vi "WSVCAP SHL Host LL SPI Write Read.vi"(0 "SPI Data [DUT Ordered]":u8[][](array[numeric]) format="%.0x", 1 "Wait Ticks":u32, 5 "Socket Mask":u16=1 format="%02x", 7 "Cycle CMD Lengths Out (bits)":u8[](array[numeric]), 9 "Cycle CMD Delay Out (ticks)":u32[](array[numeric]), 11 "error in":errorcluster) -> (4 "SPI Read Data [DUT Ordered]":u8[][](array[numeric]), 8 "Status":u8[](array[numeric]), 15 "error out":errorcluster)   [LabVIEW 2012]
uses:
  Type Defs/WSVCAP SHL Top Level Write Read State Enum.ctl
  Type Defs/WSVCAP SHL State.ctl
  Type Defs/WSVCAP SHL Top Level Control Enum.ctl
panel:
  out "Bit Array":u32[](array[numeric]) format="%.0x"
  out "Write Data":u64[](array[numeric]) format="%032b"
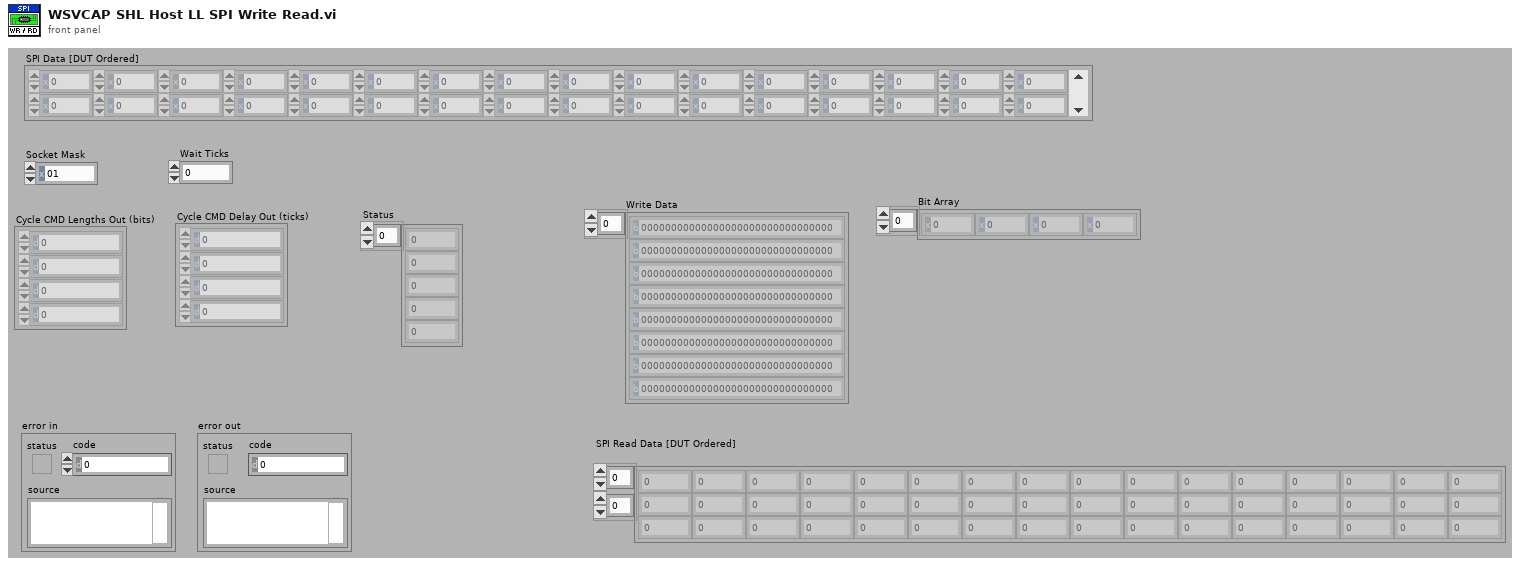
[diagram p1: front panel]
types:
  T1 = typedef "WSVCAP SHL Top Level Write Read State Enum.ctl" = enum16{"Start", "Write", "Read", "Get Status", "Wait Until Done"}
  T2 = typedef "WSVCAP SHL State.ctl" = enum8{"Idle", "Transfer Data"}
  T3 = typedef "WSVCAP SHL Top Level Control Enum.ctl" = enum16{"Start", "Cmd", "Transaction", "Wait Ticks", "Socket Mask", "Slave Address", "Sub Address", "Bytes to Write", "Bytes to Read", "Write Data", "Write Flag", "Read Data", "Read Flag", "Ack Read", "Read Status Flag", "Ack Read Status", "Status", "Cycle Count", "Stop Cycle", "Exit"}
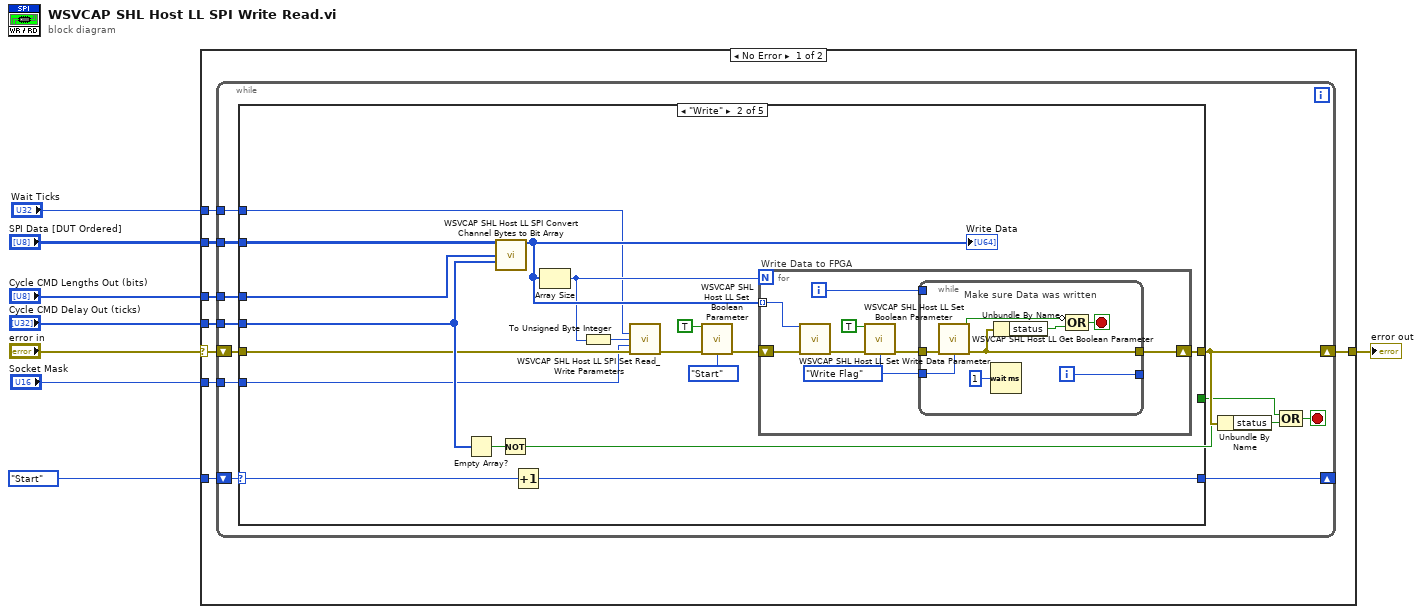
[diagram p0: block diagram]
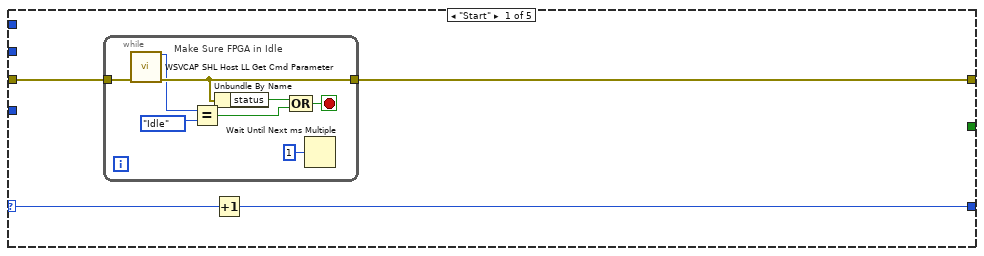
[diagram p2: hidden frame]
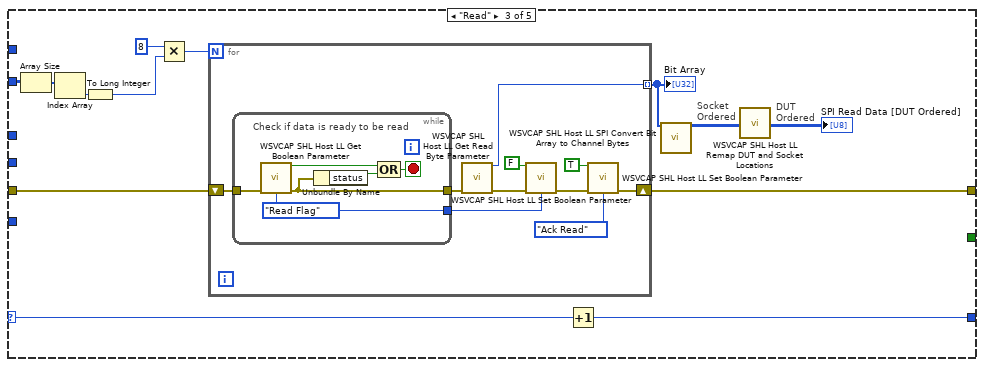
[diagram p3: hidden frame]
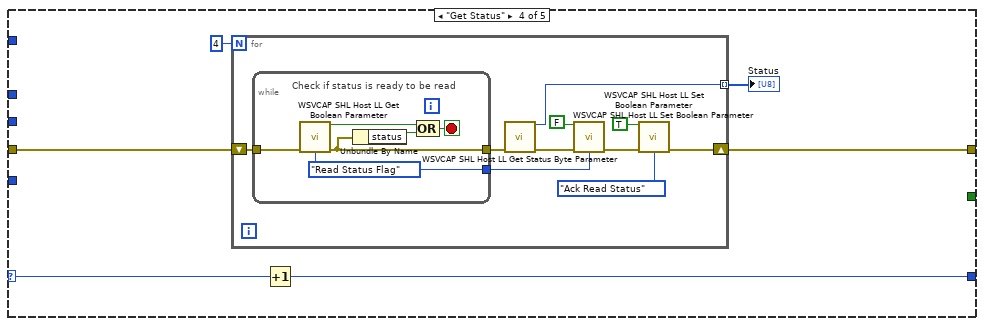
[diagram p4: hidden frame]
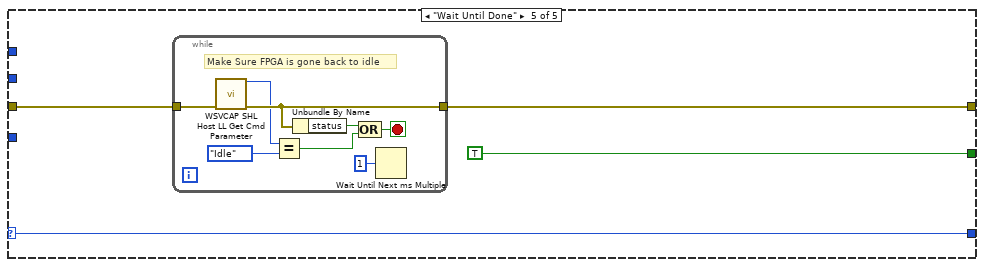
[diagram p5: hidden frame]
diagram:
  n1 = case shown="No Error" "error in" {
    selector: "error in" -> [w12 w138]
    tunnel: [w16 w138] -> w8
    tunnel: WSVCAP_SHL_Top_Level_Write_Read_State_Enum."Start" ("Write Read State") -> [w15 _]
    tunnel: "SPI Data [DUT Ordered]" -> [w14 _]
    tunnel: "Socket Mask" -> [w13 _]
    tunnel: "Cycle CMD Lengths Out (bits)" -> [w11 _]
    tunnel: "Cycle CMD Delay Out (ticks)" -> [w10 _]
    tunnel: "Wait Ticks" -> [w9 _]
    frame No Error {
      n2 = while {
        shift-right: [w27] -> w16
        shift-left: w12 -> [w28]
        shift-right: [w22] -> _
        shift-left: w15 -> [w23]
        tunnel: w14 -> [w21]
        tunnel: w13 -> [w20]
        tunnel: w11 -> [w19]
        tunnel: w10 -> [w18]
        tunnel: w9 -> [w17]
        stop <- w24 stop-if-true
        n3 = case shown="\"Write\"" w23 {
          selector: w23 -> [w31 w57 w87 w107 w127]
          tunnel: w28 -> [w32 w46 w75 w109 w129]
          tunnel: [w29 w58 w82 w108 w128] -> w27
          tunnel: [_ w51 _ _ TRUE] -> w26
          tunnel: [w30 w55 w86 w106 w127] -> w22
          tunnel: w21 -> [_ w42 w81 _ _]
          tunnel: w20 -> [_ w43 _ _ _]
          tunnel: w19 -> [_ w54 _ _ _]
          tunnel: w18 -> [_ w53 _ _ _]
          tunnel: w17 -> [_ w41 _ _ _]
          frame "Start" {
            n4 = while {
              tunnel: w32 -> [w36]
              tunnel: [w35] -> w29
              stop <- w40 stop-if-true
              # "Make Sure FPGA in Idle"
              n5 = call "WSVCAP SHL Host LL Get Cmd Parameter.vi"("error in (no error)"=w36) -> ("I2C_Cmd"=w34:T2, "error out"=w35:errorcluster)  [unwired: 13 in]
              n6 = Equal?(x=w34, y=WSVCAP_SHL_State."Idle" ("Type")) -> (x = y?=w38:bool)
              n7 = Unbundle By Name(w35) -> ("status"=w33:bool)
              n8 = Compound Arithmetic op=OR(w33, w38) -> (w40:bool)
              n9 = Wait Until Next ms Multiple(millisecond multiple=u32 1) -> ()  [unwired: 1 out]
            }
            n10 = Increment(x=w31) -> (x+1=w30:T1)
          }
          frame "Write" {
            # "Write Data to FPGA"
            n11 = Empty Array?(array=w53) -> (empty?=w52:bool)
            n12 = call "WSVCAP SHL Host LL SPI Convert Channel Bytes to Bit Array.vi"("SPI Data [DUT Ordered]"=w42, "Cycle CMD Lengths Out (bits)"=w54, "Cycle CMD Delay Out (ticks)"=w53) -> ("Write Data"=w56:u64[])  [unwired: 12 in]
            "Write Data" <- w56
            n13 = Not(x=w52) -> (.not. x?=w51:bool)
            n14 = Increment(x=w57) -> (x+1=w55:T1)
            n15 = Array Size(array=w56) -> (size(s)=w44:i32)
            n16 = To Unsigned Byte Integer(number=w44) -> (unsigned 8bit integer=w47:u8)
            n17 = call "WSVCAP SHL Host LL SPI Set Read_Write Parameters.vi"("Wait Ticks"=w41, "Elements to Transfer"=w47, "Socket Mask [U16]"=w43, "error in (no error)"=w46) -> ("error out"=w50:errorcluster)  [unwired: 11 in]
            n18 = call "WSVCAP SHL Host LL Set Boolean Parameter.vi"("Boolean In"=TRUE, "error in (no error)"=w50, "FPGA Top Level Control"=WSVCAP_SHL_Top_Level_Control_Enum."Start") -> ("error out"=w45:errorcluster)  [unwired: 12 in]
            n19 = for {
              N: w44 -> [_]
              shift-right: [w66] -> w58
              shift-left: w45 -> [w65]
              tunnel: w56 -> [w64] mode=indexing
              i -> [w59]
              w60 = WSVCAP_SHL_Top_Level_Control_Enum."Write Flag" ("FPGA Top Level Control")
              n20 = call "WSVCAP SHL Host LL Set Write Data Parameter.vi"("Write Byte In"=w64, "error in (no error)"=w65) -> ("error out"=w63:errorcluster)  [unwired: 13 in]
              n21 = call "WSVCAP SHL Host LL Set Boolean Parameter.vi"("Boolean In"=TRUE, "error in (no error)"=w63, "FPGA Top Level Control"=w60) -> ("error out"=w61:errorcluster)  [unwired: 12 in]
              n22 = while {
                tunnel: w61 -> [w72]
                tunnel: [w71] -> w66
                tunnel: w60 -> [w69]
                tunnel: w59 -> [_]
                tunnel: [w67] -> _
                i -> [w67]
                stop <- w74 stop-if-true
                # "Make sure Data was written"
                n23 = call "WSVCAP SHL Host LL Get Boolean Parameter.vi"("error in (no error)"=w72, "FPGA Top Level Control"=w69) -> ("Boolean Out"=w70:bool, "error out"=w71:errorcluster)  [unwired: 12 in]
                n24 = Wait (ms)(milliseconds to wait=u32 1) -> ()  [unwired: 1 out]
                n25 = Unbundle By Name(w71) -> ("status"=w68:bool)
                n26 = Compound Arithmetic op=OR(invert w70, w68) -> (w74:bool)
              }
            }
          }
          frame "Read" {
            # "DUT\nOrdered"
            # "Socket\nOrdered"
            n27 = Array Size(array=w81) -> (size(s)=w80:i32[])
            n28 = Index Array(array=w80) -> (element=w79:i32)  [unwired: 1 in]
            n29 = To Long Integer(number=w79) -> (32bit integer=w76:i32)
            n30 = Multiply(x=8, y=w76) -> (x*y=w84:i32)
            n31 = for {
              N: w84 -> [_]
              shift-right: [w94] -> w82
              shift-left: w75 -> [w97]
              tunnel: [w88] -> w85 mode=indexing
              n32 = while {
                tunnel: w97 -> [w101]
                tunnel: [w100] -> w96
                tunnel: [w98] -> w93
                stop <- w103 stop-if-true
                w98 = WSVCAP_SHL_Top_Level_Control_Enum."Read Flag" ("FPGA Top Level Control")
                # "Check if data is ready to be read"
                n33 = call "WSVCAP SHL Host LL Get Boolean Parameter.vi"("error in (no error)"=w101, "FPGA Top Level Control"=w98) -> ("Boolean Out"=w102:bool, "error out"=w100:errorcluster)  [unwired: 12 in]
                n34 = Unbundle By Name(w100) -> ("status"=w99:bool)
                n35 = Compound Arithmetic op=OR(w102, w99) -> (w103:bool)
              }
              n36 = call "WSVCAP SHL Host LL Get Read Byte Parameter.vi"("error in (no error)"=w96) -> ("Read Data In"=w88:u64, "error out"=w95:errorcluster)  [unwired: 13 in]
              n37 = call "WSVCAP SHL Host LL Set Boolean Parameter.vi"("Boolean In"=FALSE ("Read Flag"), "error in (no error)"=w95, "FPGA Top Level Control"=w93) -> ("error out"=w89:errorcluster)  [unwired: 12 in]
              n38 = call "WSVCAP SHL Host LL Set Boolean Parameter.vi"("Boolean In"=TRUE ("Write Flag"), "error in (no error)"=w89, "FPGA Top Level Control"=WSVCAP_SHL_Top_Level_Control_Enum."Ack Read") -> ("error out"=w94:errorcluster)  [unwired: 12 in]
            }
            "Bit Array" <- w85
            n39 = Increment(x=w87) -> (x+1=w86:T1)
            n40 = call "WSVCAP SHL Host LL SPI Convert Bit Array to Channel Bytes.vi"("Bit Array"=w85) -> ("SPI Read Data [Socket Ordered]"=w78:u8[][])  [unwired: 14 in]
            n41 = call "WSVCAP SHL Host LL Remap DUT and Socket Locations.vi"("C1 Socket Ordered Data In"=w78) -> ("C1 DUT Ordered Data Out"=→"SPI Read Data [DUT Ordered]":u8[][])  [unwired: 13 in, 5 out]
          }
          frame "Get Status" {
            n42 = for {
              N: 4 -> [_]
              shift-right: [w118] -> w108
              shift-left: w109 -> [w119]
              tunnel: [w110] -> w104 mode=indexing
              n43 = while {
                tunnel: w119 -> [w123]
                tunnel: [w122] -> w117
                tunnel: [w120] -> w115
                stop <- w125 stop-if-true
                w120 = WSVCAP_SHL_Top_Level_Control_Enum."Read Status Flag" ("FPGA Top Level Control")
                # "Check if status is ready to be read"
                n44 = call "WSVCAP SHL Host LL Get Boolean Parameter.vi"("error in (no error)"=w123, "FPGA Top Level Control"=w120) -> ("Boolean Out"=w124:bool, "error out"=w122:errorcluster)  [unwired: 12 in]
                n45 = Unbundle By Name(w122) -> ("status"=w121:bool)
                n46 = Compound Arithmetic op=OR(w124, w121) -> (w125:bool)
              }
              n47 = call "WSVCAP SHL Host LL Get Status Byte Parameter.vi"("error in (no error)"=w117) -> ("I2C Status Byte"=w110:u8, "error out"=w116:errorcluster)  [unwired: 13 in]
              n48 = call "WSVCAP SHL Host LL Set Boolean Parameter.vi"("Boolean In"=FALSE ("Read Flag"), "error in (no error)"=w116, "FPGA Top Level Control"=w115) -> ("error out"=w111:errorcluster)  [unwired: 12 in]
              n49 = call "WSVCAP SHL Host LL Set Boolean Parameter.vi"("Boolean In"=TRUE ("Write Flag"), "error in (no error)"=w111, "FPGA Top Level Control"=WSVCAP_SHL_Top_Level_Control_Enum."Ack Read Status") -> ("error out"=w118:errorcluster)  [unwired: 12 in]
            }
            "Status" <- w104
            n50 = Increment(x=w107) -> (x+1=w106:T1)
          }
          frame "Wait Until Done" {
            n51 = while {
              tunnel: w129 -> [w132]
              tunnel: [w131] -> w128
              stop <- w134 stop-if-true
              # "Make Sure FPGA is gone back to idle"
              n52 = call "WSVCAP SHL Host LL Get Cmd Parameter.vi"("error in (no error)"=w132) -> ("I2C_Cmd"=w130:T2, "error out"=w131:errorcluster)  [unwired: 13 in]
              n53 = Equal?(x=w130, y=WSVCAP_SHL_State."Idle") -> (x = y?=w135:bool)
              n54 = Unbundle By Name(w131) -> ("status"=w136:bool)
              n55 = Compound Arithmetic op=OR(w136, w135) -> (w134:bool)
              n56 = Wait Until Next ms Multiple(millisecond multiple=u32 1) -> ()  [unwired: 1 out]
            }
          }
        }
        n57 = Unbundle By Name(w27) -> ("status"=w25:bool)
        n58 = Compound Arithmetic op=OR(w26, w25) -> (w24:bool)
      }
    }
    frame Error {
    }
  }
  "error out" <- w8
